vi "Init A.vi"(8 "error in (no error)":errorcluster, 10 "Boolean":bool, 11 "DA Child A in":refnum<class "DA Child A.lvclass">) -> (0 "error out":errorcluster, 3 "DA Child A out":refnum<class "DA Child A.lvclass">)   [LabVIEW 2020, in "Display As.lvlib" / "DA Child A.lvclass"]
uses:
  DA Child A.lvclass
  DA Child A.lvclass/DA Child A.ctl
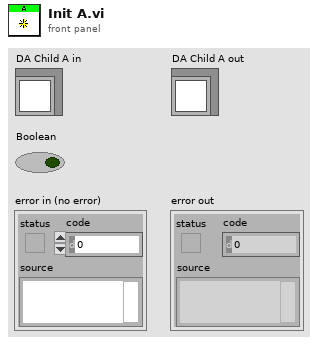
[diagram p1: front panel]
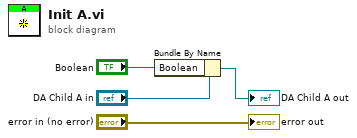
[diagram p0: block diagram]
diagram:
  n1 = Bundle By Name(cluster="DA Child A in", "Boolean"="Boolean") -> (→"DA Child A out":refnum<class "DA Child A.lvclass">)
  "error out" <- "error in (no error)"
